vi "3_3.vi"() -> ()   [LabVIEW 2012]
panel:
  in  "51-61":bool
  in  "1-11":bool
  in  "0-100":bool
  out "3":dbl[][][](array[numeric])
  out "2":dbl[][](array[numeric])
  out "1":dbl[](array[numeric])
  in  "0-10":bool
  in  "stop":bool
  in  "0-1":bool
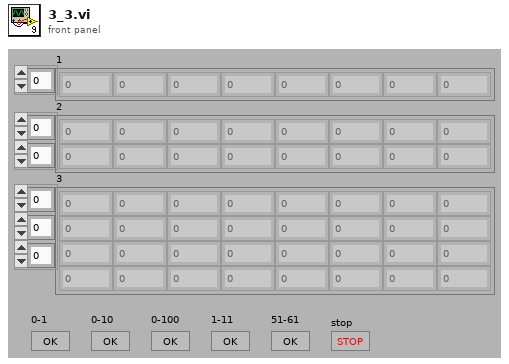
[diagram p1: front panel]
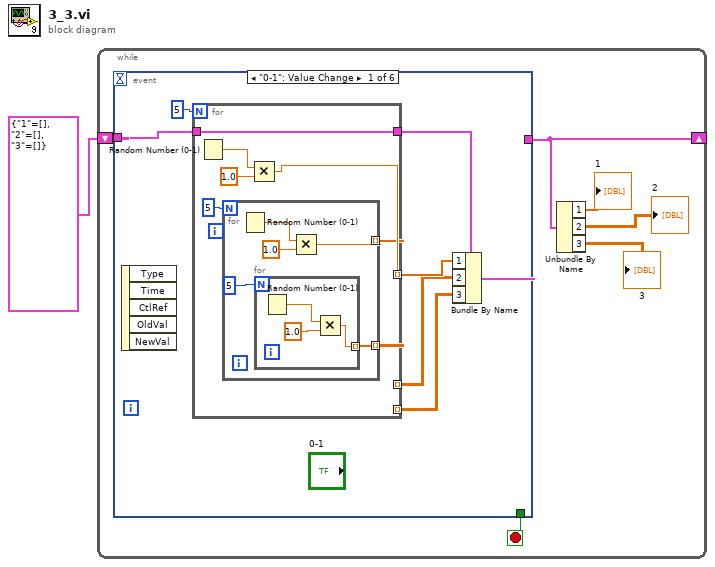
[diagram p0: block diagram]
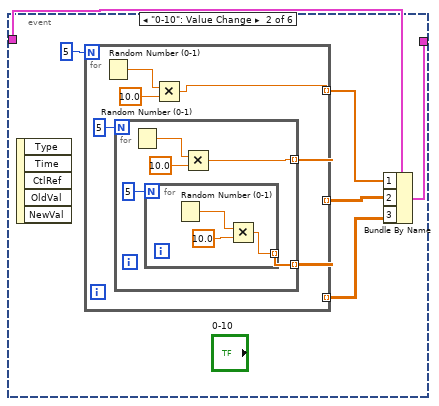
[diagram p2: hidden frame]
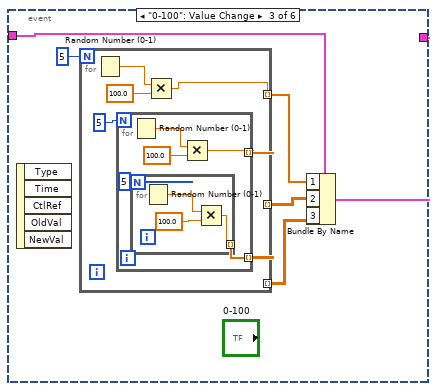
[diagram p3: hidden frame]
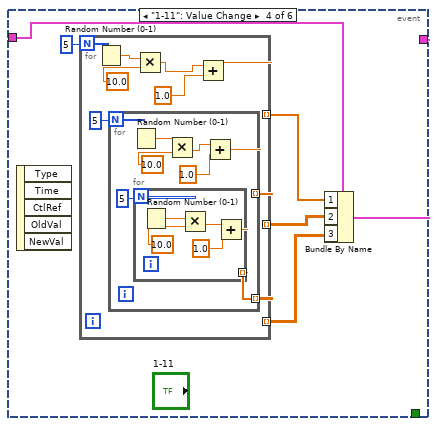
[diagram p4: hidden frame]
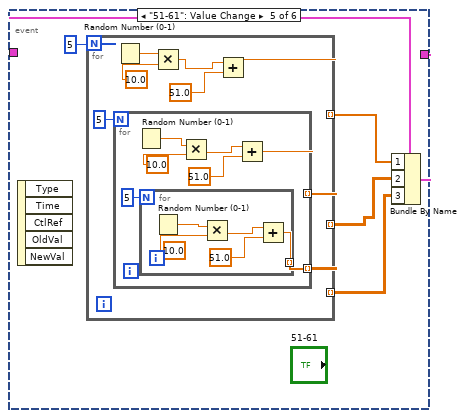
[diagram p5: hidden frame]
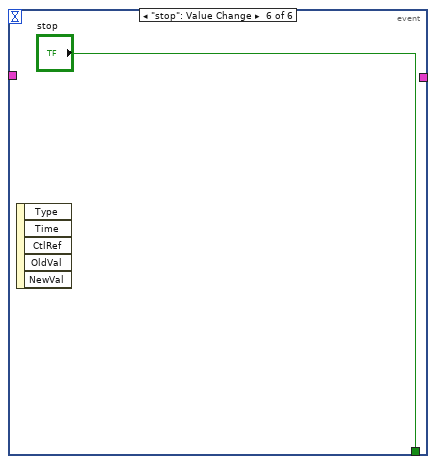
[diagram p6: hidden frame]
diagram:
  n1 = while {
    shift-right: [w5] -> _
    shift-left: cluster{"1":dbl[], "2":dbl[][], "3":dbl[][][]} {"1"=[], "2"=[], "3"=[]} -> [w6]
    stop <- w7 stop-if-true
    n2 = event shown="[0] \"0-1\": Value Change" {
      selector: _ -> [_ _ _ _ _ _]
      dyn-events: _ -> [_ _ _ _ _ _]
      timeout: _ -> [_ _ _ _ _ _]
      tunnel: [_ _ _ _ _ "stop"] -> w7
      tunnel: w6 -> [w13 w34 w51 w71 w97 _]
      tunnel: [w8 w30 w50 w70 w96 _] -> w5
      event "0-1": Value Change {
        n3 = event-data() -> ()  [unwired: 1 in, 5 out]
        n4 = for {
          N: 5 -> [_]
          tunnel: [w21] -> w11 mode=indexing
          tunnel: [w17] -> w10 mode=indexing
          tunnel: [w16] -> w9 mode=indexing
          tunnel: w13 -> [w15]
          tunnel: [w15] -> w12
          n5 = Random Number (0-1)() -> (number: 0 to 1=w20:dbl)
          n6 = for {
            N: 5 -> [_]
            tunnel: [w26] -> w17 mode=indexing
            tunnel: [w22] -> w16 mode=indexing
            n7 = Random Number (0-1)() -> (number: 0 to 1=w25:dbl)
            n8 = for {
              N: 5 -> [_]
              tunnel: [w29] -> w22 mode=indexing
              n9 = Random Number (0-1)() -> (number: 0 to 1=w28:dbl)
              n10 = Multiply(x=w28, y=1.0) -> (x*y=w29:dbl)
            }
            n11 = Multiply(x=w25, y=1.0) -> (x*y=w26:dbl)
          }
          n12 = Multiply(x=w20, y=1.0) -> (x*y=w21:dbl)
        }
        n13 = Bundle By Name(cluster=w12, "1"=w11, "2"=w10, "3"=w9) -> (w8:cluster{"1":dbl[], "2":dbl[][], "3":dbl[][][]})
      }
      event "0-10": Value Change {
        n14 = event-data() -> ()  [unwired: 1 in, 5 out]
        n15 = for {
          N: 5 -> [_]
          tunnel: [w41] -> w33 mode=indexing
          tunnel: [w37] -> w32 mode=indexing
          tunnel: [w36] -> w31 mode=indexing
          n16 = Random Number (0-1)() -> (number: 0 to 1=w40:dbl)
          n17 = for {
            N: 5 -> [_]
            tunnel: [w46] -> w37 mode=indexing
            tunnel: [w42] -> w36 mode=indexing
            n18 = Random Number (0-1)() -> (number: 0 to 1=w45:dbl)
            n19 = for {
              N: 5 -> [_]
              tunnel: [w49] -> w42 mode=indexing
              n20 = Random Number (0-1)() -> (number: 0 to 1=w48:dbl)
              n21 = Multiply(x=w48, y=10.0) -> (x*y=w49:dbl)
            }
            n22 = Multiply(x=w45, y=10.0) -> (x*y=w46:dbl)
          }
          n23 = Multiply(x=w40, y=10.0) -> (x*y=w41:dbl)
        }
        n24 = Bundle By Name(cluster=w34, "1"=w33, "2"=w32, "3"=w31) -> (w30:cluster{"1":dbl[], "2":dbl[][], "3":dbl[][][]})
      }
      event "0-100": Value Change {
        n25 = event-data() -> ()  [unwired: 1 in, 5 out]
        n26 = for {
          N: 5 -> [_]
          tunnel: [w61] -> w54 mode=indexing
          tunnel: [w57] -> w53 mode=indexing
          tunnel: [w56] -> w52 mode=indexing
          n27 = Random Number (0-1)() -> (number: 0 to 1=w60:dbl)
          n28 = for {
            N: 5 -> [_]
            tunnel: [w66] -> w57 mode=indexing
            tunnel: [w62] -> w56 mode=indexing
            n29 = Random Number (0-1)() -> (number: 0 to 1=w65:dbl)
            n30 = for {
              N: 5 -> [_]
              tunnel: [w69] -> w62 mode=indexing
              n31 = Random Number (0-1)() -> (number: 0 to 1=w68:dbl)
              n32 = Multiply(x=w68, y=100.0) -> (x*y=w69:dbl)
            }
            n33 = Multiply(x=w65, y=100.0) -> (x*y=w66:dbl)
          }
          n34 = Multiply(x=w60, y=100.0) -> (x*y=w61:dbl)
        }
        n35 = Bundle By Name(cluster=w51, "1"=w54, "2"=w53, "3"=w52) -> (w50:cluster{"1":dbl[], "2":dbl[][], "3":dbl[][][]})
      }
      event "1-11": Value Change {
        n36 = event-data() -> ()  [unwired: 1 in, 5 out]
        n37 = for {
          N: 5 -> [_]
          tunnel: [w76] -> w74 mode=indexing
          tunnel: [w82] -> w73 mode=indexing
          tunnel: [w81] -> w72 mode=indexing
          n38 = Random Number (0-1)() -> (number: 0 to 1=w80:dbl)
          n39 = for {
            N: 5 -> [_]
            tunnel: [w84] -> w82 mode=indexing
            tunnel: [w89] -> w81 mode=indexing
            n40 = Random Number (0-1)() -> (number: 0 to 1=w85:dbl)
            n41 = for {
              N: 5 -> [_]
              tunnel: [w91] -> w89 mode=indexing
              n42 = Random Number (0-1)() -> (number: 0 to 1=w95:dbl)
              n43 = Multiply(x=w95, y=10.0 ("x")) -> (x*y=w92:dbl)
              n44 = Add(x=w92, y=1.0) -> (x+y=w91:dbl)
            }
            n45 = Multiply(x=w85, y=10.0 ("x")) -> (x*y=w88:dbl)
            n46 = Add(x=w88, y=1.0) -> (x+y=w84:dbl)
          }
          n47 = Multiply(x=w80, y=10.0 ("x")) -> (x*y=w77:dbl)
          n48 = Add(x=w77, y=1.0) -> (x+y=w76:dbl)
        }
        n49 = Bundle By Name(cluster=w71, "1"=w74, "2"=w73, "3"=w72) -> (w70:cluster{"1":dbl[], "2":dbl[][], "3":dbl[][][]})
      }
      event "51-61": Value Change {
        n50 = event-data() -> ()  [unwired: 1 in, 5 out]
        n51 = for {
          N: 5 -> [_]
          tunnel: [w102] -> w100 mode=indexing
          tunnel: [w108] -> w99 mode=indexing
          tunnel: [w107] -> w98 mode=indexing
          n52 = for {
            N: 5 -> [_]
            tunnel: [w110] -> w108 mode=indexing
            tunnel: [w115] -> w107 mode=indexing
            n53 = Random Number (0-1)() -> (number: 0 to 1=w111:dbl)
            n54 = for {
              N: 5 -> [_]
              tunnel: [w117] -> w115 mode=indexing
              n55 = Random Number (0-1)() -> (number: 0 to 1=w121:dbl)
              n56 = Multiply(x=w121, y=10.0 ("x")) -> (x*y=w118:dbl)
              n57 = Add(x=w118, y=51.0) -> (x+y=w117:dbl)
            }
            n58 = Multiply(x=w111, y=10.0 ("x")) -> (x*y=w114:dbl)
            n59 = Add(x=w114, y=51.0) -> (x+y=w110:dbl)
          }
          n60 = Random Number (0-1)() -> (number: 0 to 1=w106:dbl)
          n61 = Multiply(x=w106, y=10.0 ("x")) -> (x*y=w103:dbl)
          n62 = Add(x=w103, y=51.0) -> (x+y=w102:dbl)
        }
        n63 = Bundle By Name(cluster=w97, "1"=w100, "2"=w99, "3"=w98) -> (w96:cluster{"1":dbl[], "2":dbl[][], "3":dbl[][][]})
      }
      event "stop": Value Change {
        n64 = event-data() -> ()  [unwired: 1 in, 5 out]
      }
    }
    n65 = Unbundle By Name(w5) -> ("1"=→"1":dbl[], "2"=→"2":dbl[][], "3"=→"3":dbl[][][])
  }
